vi "acq_eeg_read.vi"(7 "Marker Queue":refnum<queue>, 8 "error in (no error)":errorcluster, 10 "variant in":variant, 11 "eeg_device":T1) -> (0 "error out":errorcluster, 1 "Next Acq State":string, 2 "Variant out":variant, 3 "eeg samples":dbl[][](array[numeric]), 5 "Marker Queue Out":refnum<queue>)   [LabVIEW 2013]
uses:
  <vilib>/NIOSC/Address Space Node.ctl
  gui/type_def/device.ctl
  <vilib>/NI/Emotiv Toolkit/Emotiv Task.lvclass
  <vilib>/NI/Emotiv Toolkit/Utilities/EE DataChannels_enum.ctl
  <vilib>/OpenBCI/Comm Protocol/Control Def/openbci_device.ctl
  <vilib>/OpenBCI/Comm Protocol/Control Def/channel_count.ctl
  gui/type_def/file_stream.ctl
  <vilib>/NIOSC/Argument to Float32 Data.vi
  <vilib>/NIOSC/Generate Error.vi
  <vilib>/NI/LabVIEW - NeuroSky Driver/NeuroSky Driver/ThinkGear Read/ThinkGear MultiSample Read Raw.vi
  <vilib>/NIOSC/NI_OSC.lvlib
  <vilib>/NI/LabVIEW - NeuroSky Driver/NeuroSky Driver.lvlib
panel:
  out "Livesign Msg":bool
  out "ECG Chart":u32[](graph)
  out "Acc Chart":dbl[][](graph)
  out "Respiration Chart":u32[](graph)
  in  "NeuroSky Task Out":T2
  in  "muse cluster out":T4
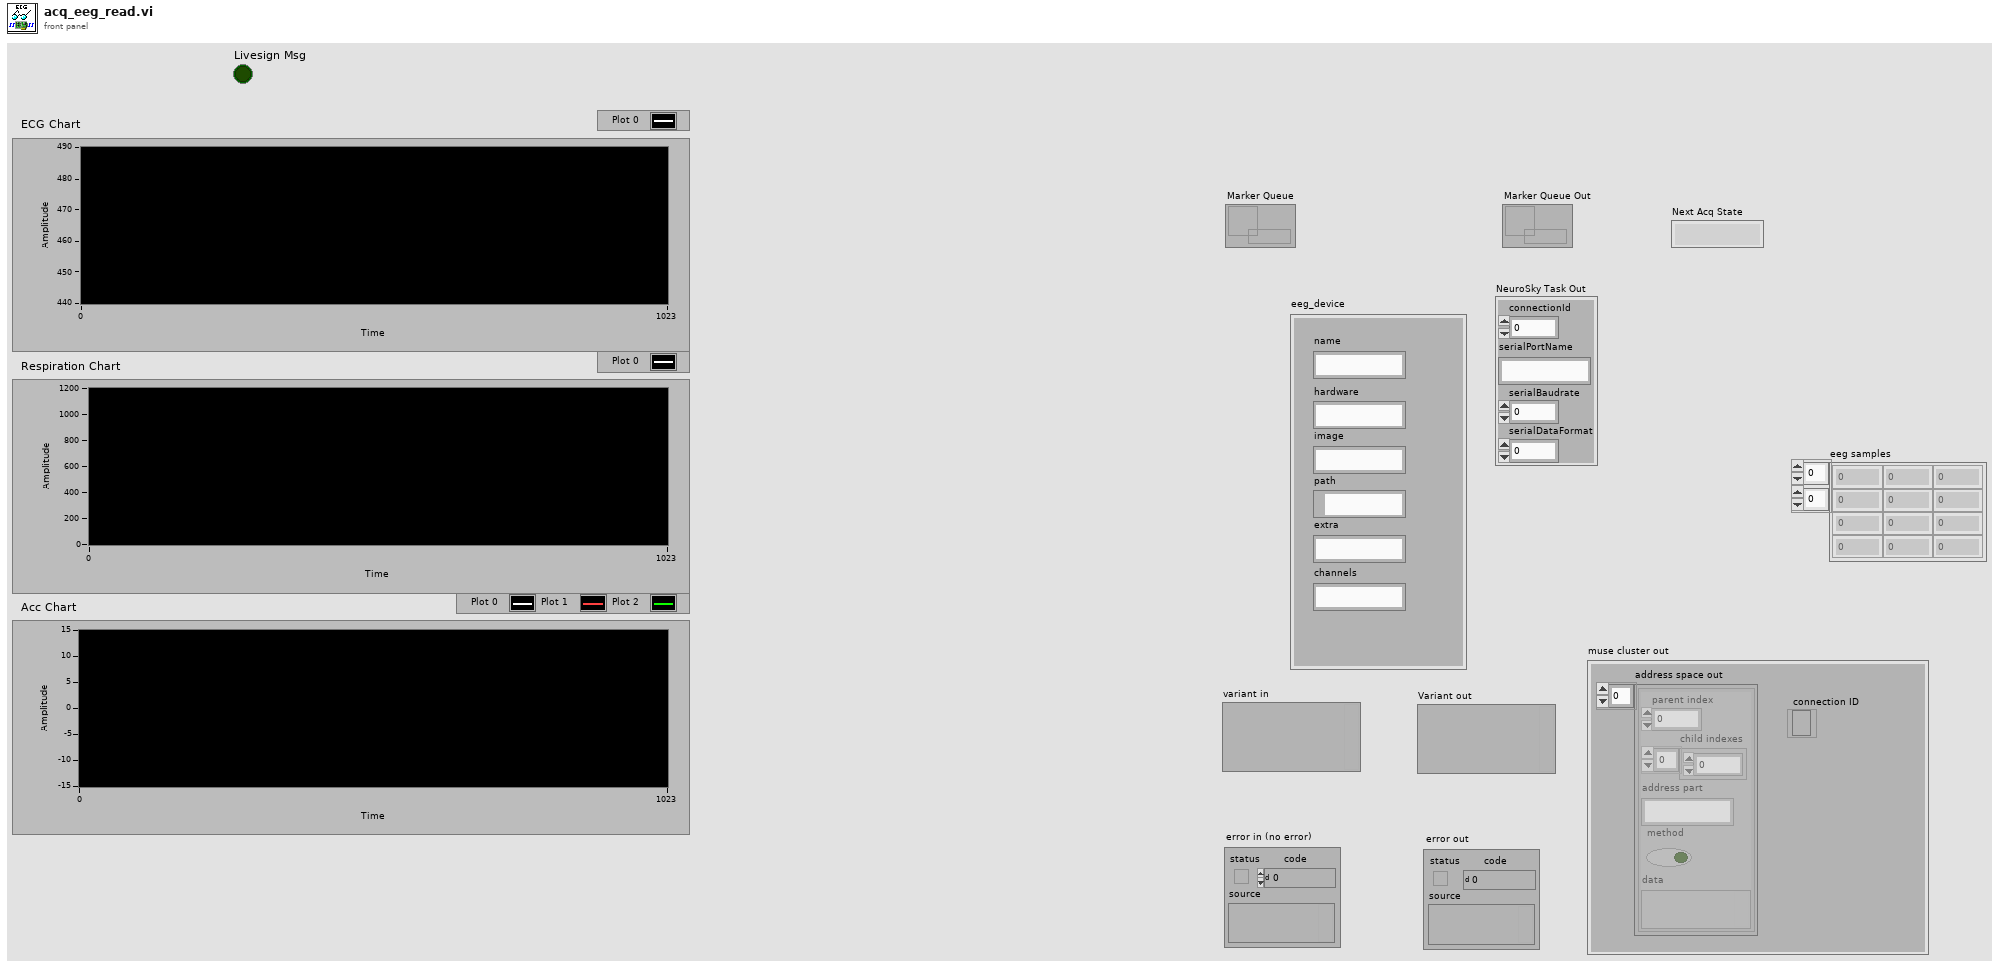
[diagram p1: front panel]
types:
  T1 = typedef "device.ctl" = cluster{"name":string, "hardware":string, "image":string, "path":path, "extra":string, "channels":string}
  T2 = cluster{"connectionId":i32, "serialPortName":string, "serialBaudrate":i32, "serialDataFormat":i32}
  T3 = typedef "NI_OSC.lvlib/Address Space Node.ctl" = cluster{"parent index":i32, "child indexes":i32[], "address part":string, "method":bool, "data":variant}
  T4 = cluster{"address space out":T3[], "connection ID":refnum<k5>}
  T5 = typedef "Emotiv Task.lvclass/EE DataChannels_enum.ctl" = enum8{"ED_COUNTER", "ED_INTERPOLATED", "ED_RAW_CQ", "ED_AF3", "ED_F7", "ED_F3", "ED_FC5", "ED_T7", "ED_P7", "ED_O1", "ED_O2", "ED_P8", "ED_T8", "ED_FC6", "ED_F4", "ED_F8", "ED_AF4", "ED_GYROX", "ED_GYROY", "ED_TIMESTAMP", "ED_ES_TIMESTAMP", "ED_FUNC_ID", "ED_FUNC_VALUE", "ED_MARKER", "ED_SYNC_SIGNAL"}
  T6 = typedef "openbci_device.ctl" = cluster{"COM port":refnum<visa-resource-name>, "n_ch (8)":T7, "delay_tx":u32}
  T7 = typedef "channel_count.ctl" = enum16{"8 Channels", "16 Channels"}
  T8 = typedef "file_stream.ctl" = cluster{"timestamp":timestamp, "data (2D array)":dbl[][], "Reading?":bool}
  T9 = typedef "NI_OSC.lvlib/Method Dispatching Info.ctl" = cluster{"method address":string, "message":string, "message timetag":u64, "data":variant}
  T10 = typedef "NI_OSC.lvlib/Argument.ctl" = cluster{"argument":string, "type tag":string}
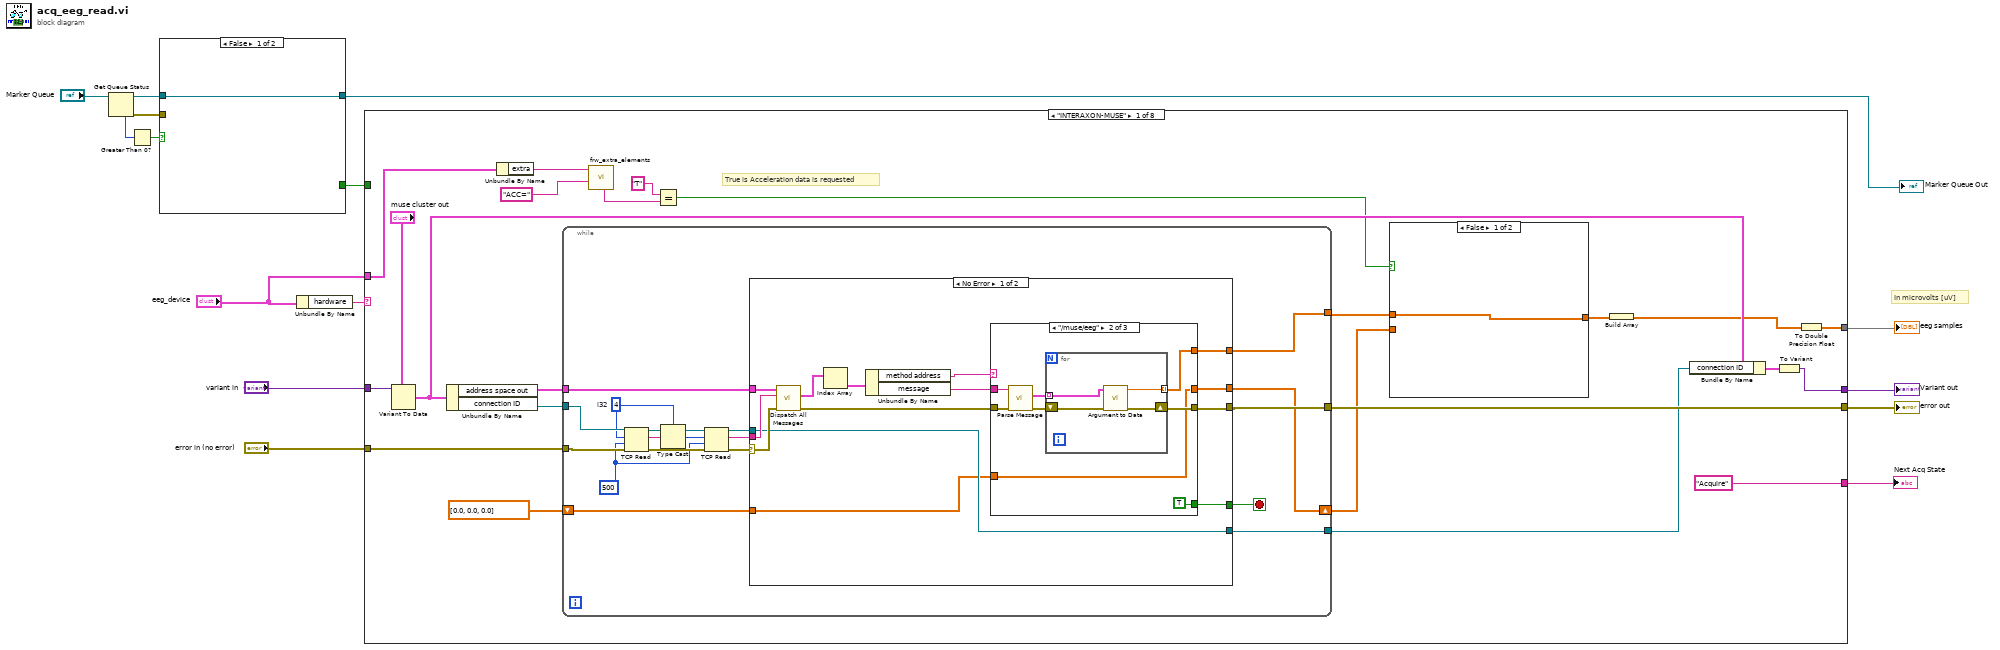
[diagram p0: block diagram]
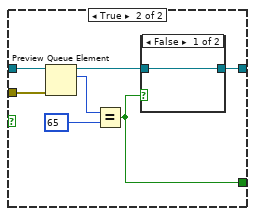
[diagram p2: hidden frame]
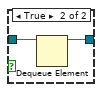
[diagram p3: hidden frame]
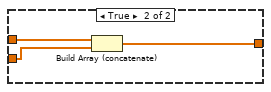
[diagram p4: hidden frame]
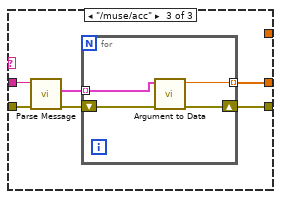
[diagram p6: hidden frame]
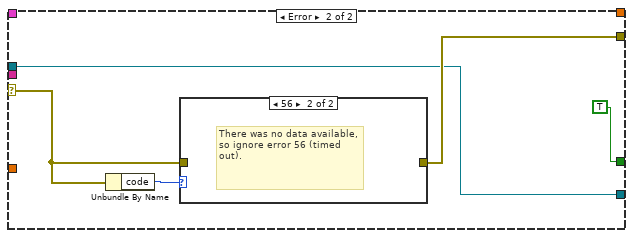
[diagram p7: hidden frame]
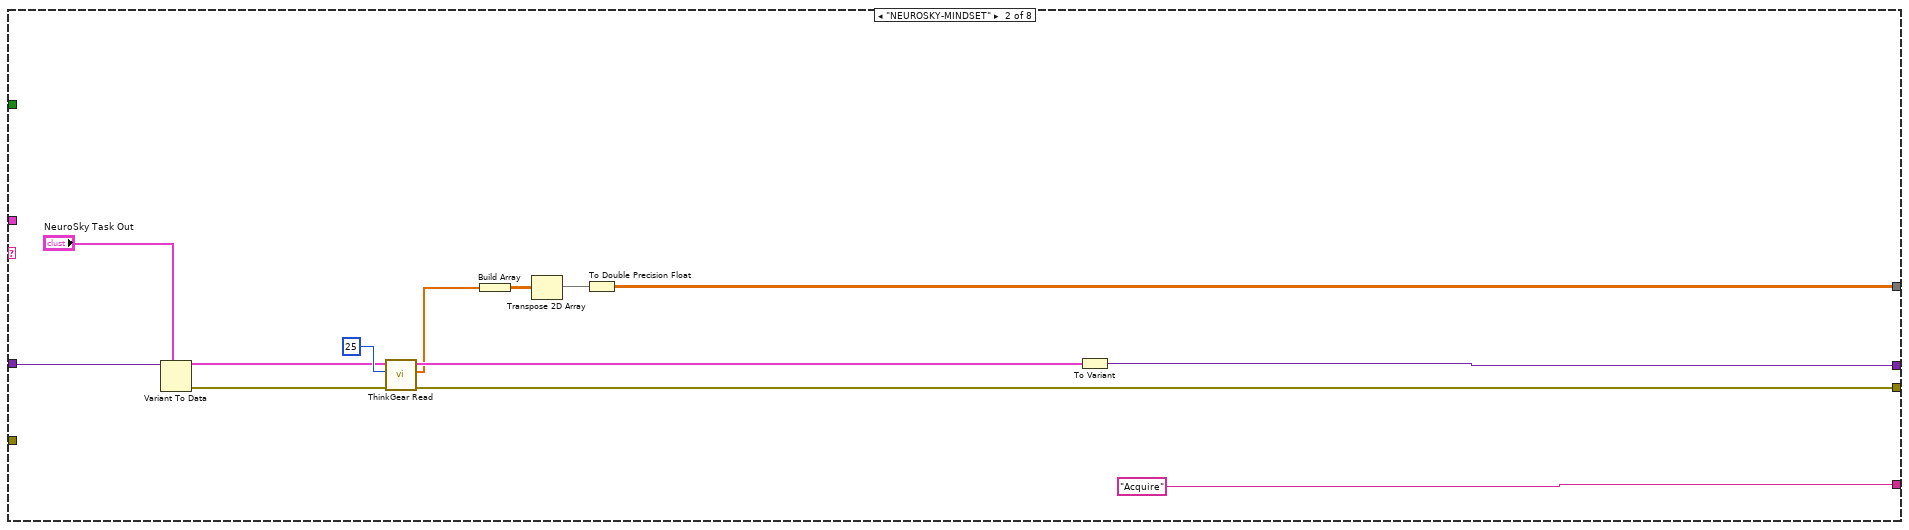
[diagram p9: hidden frame]
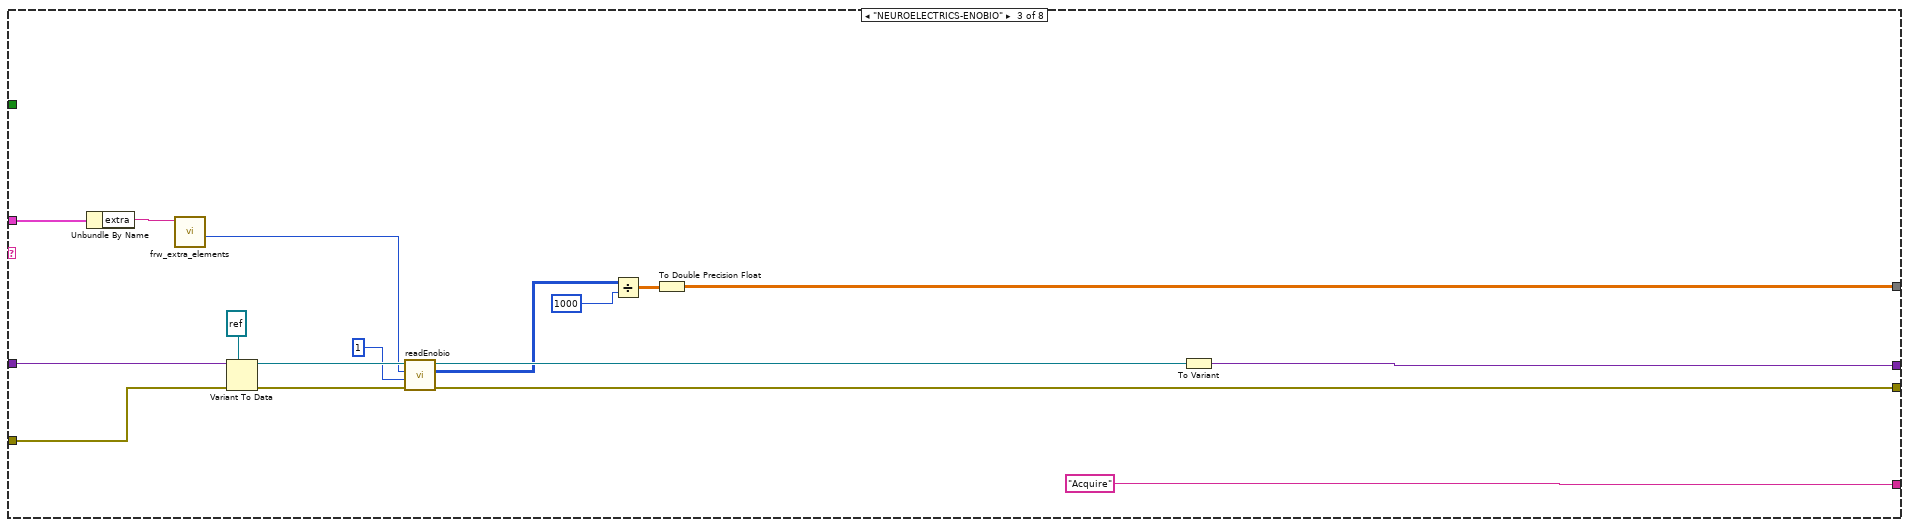
[diagram p10: hidden frame]
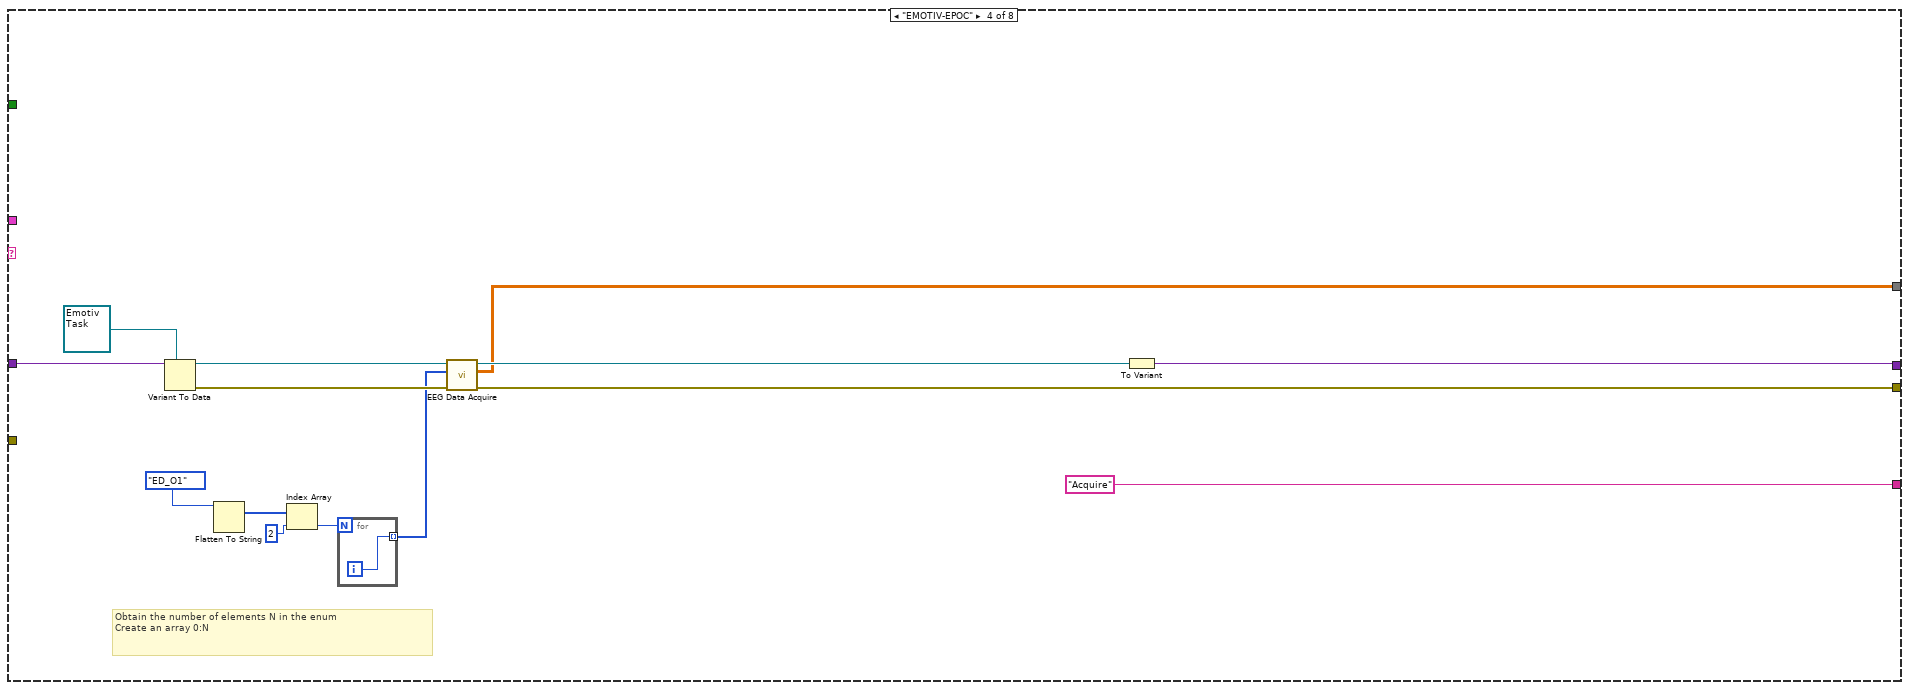
[diagram p11: hidden frame]
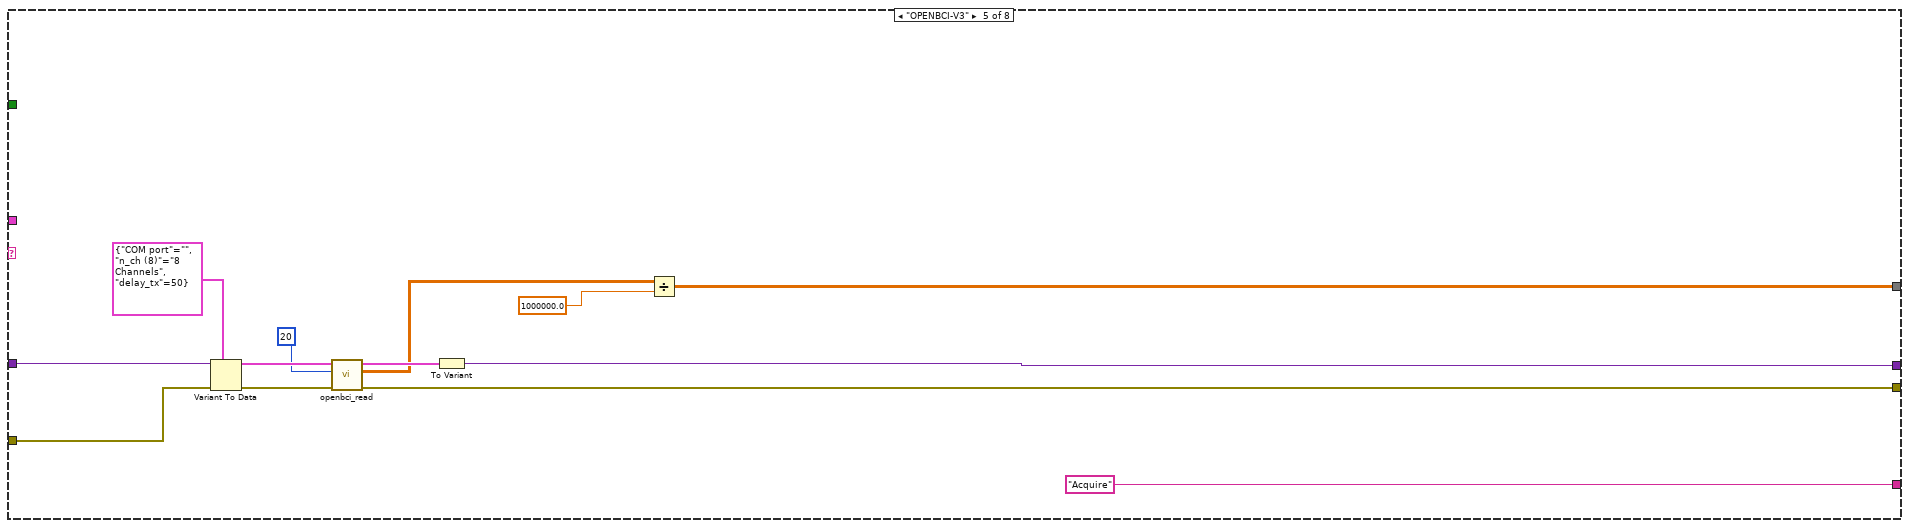
[diagram p12: hidden frame]
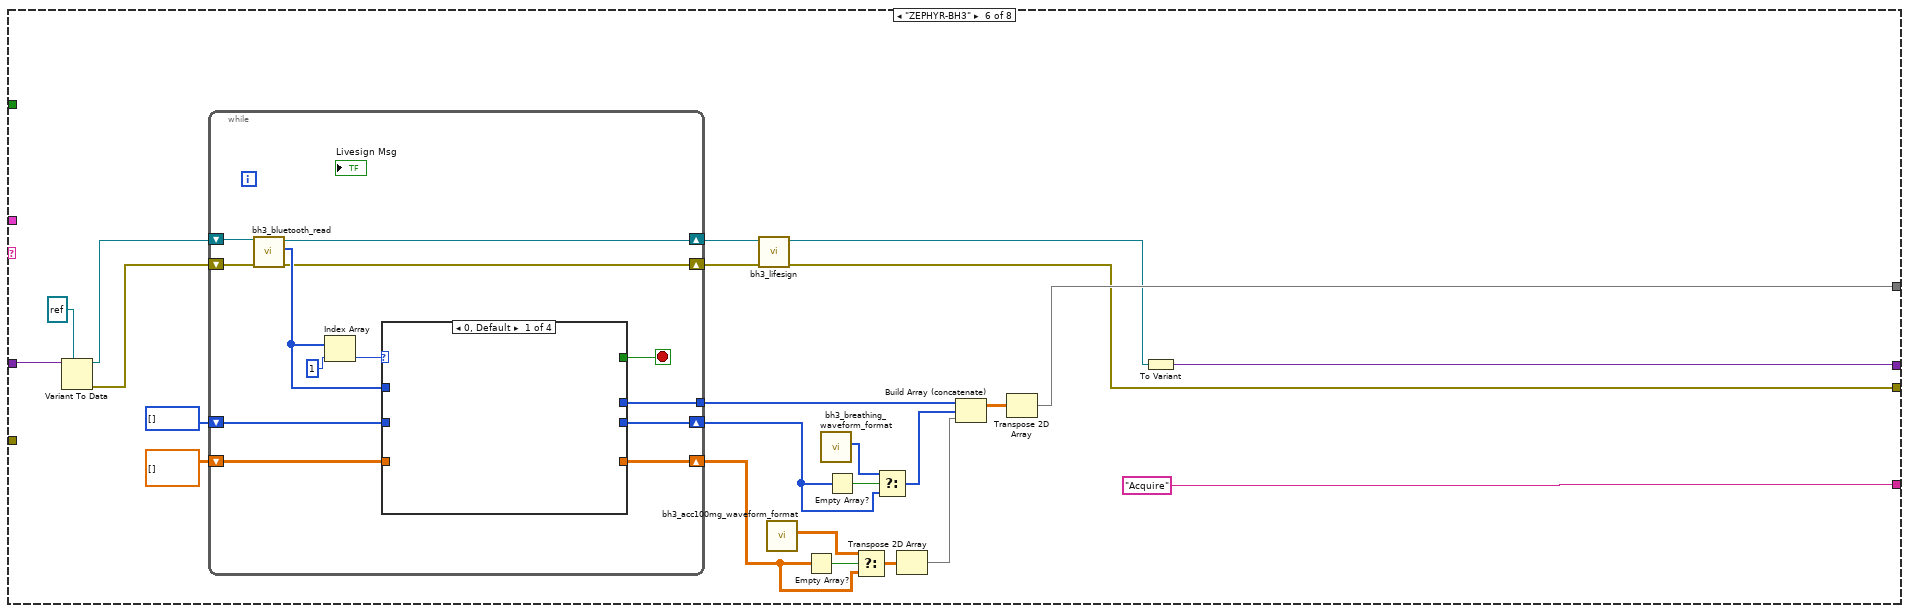
[diagram p13: hidden frame]
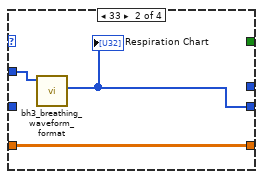
[diagram p14: hidden frame]
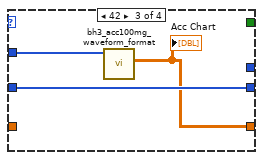
[diagram p15: hidden frame]
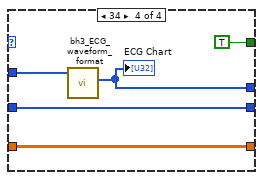
[diagram p16: hidden frame]
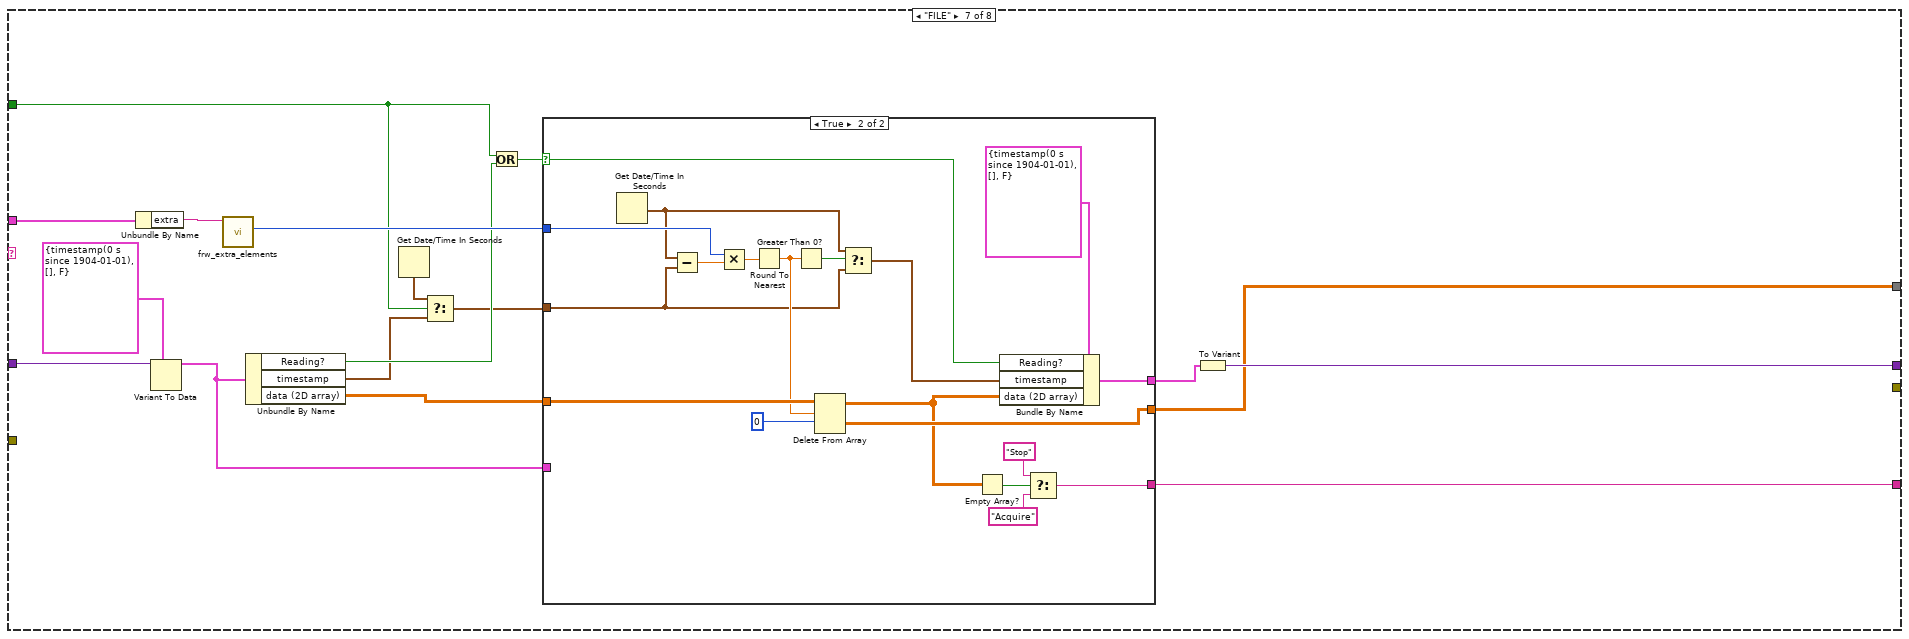
[diagram p17: hidden frame]
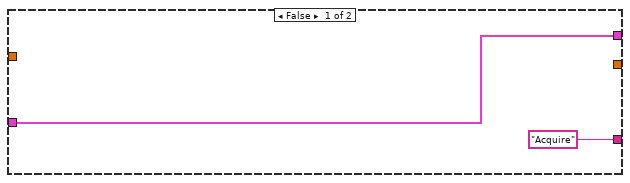
[diagram p18: hidden frame]
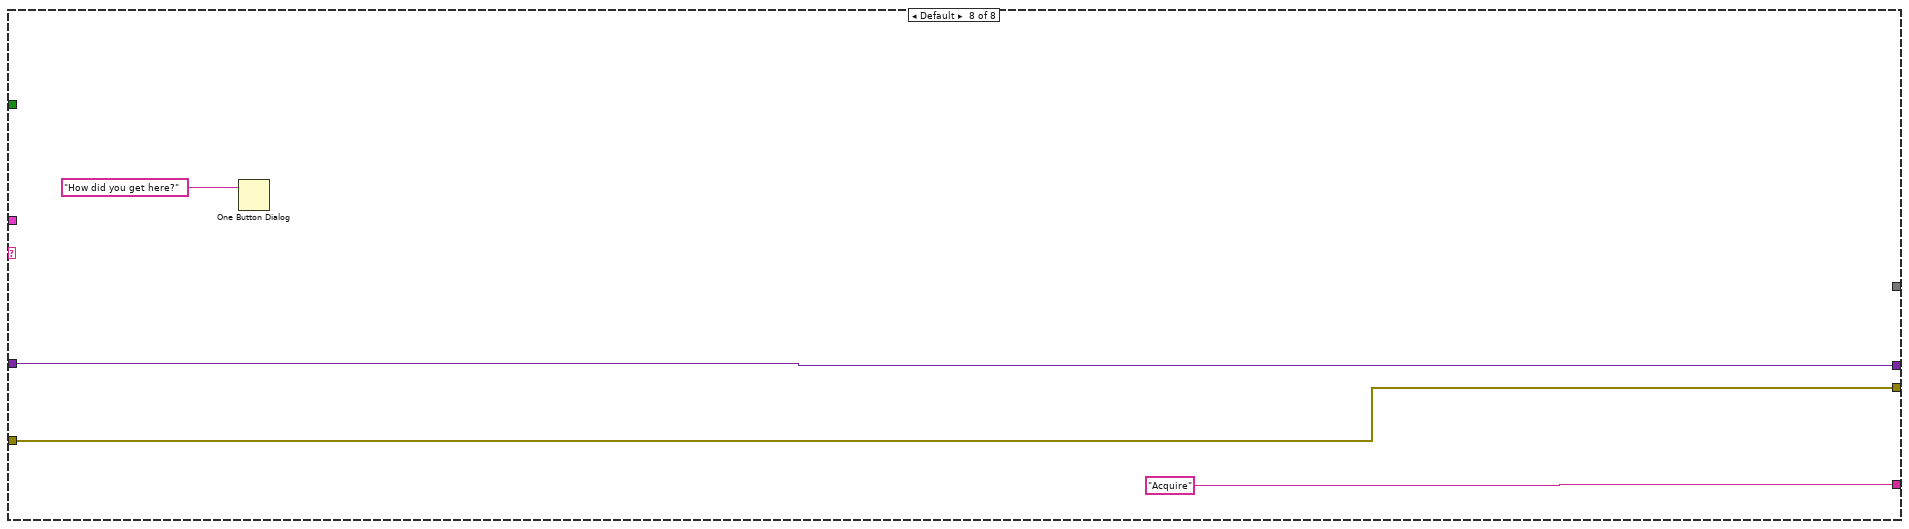
[diagram p19: hidden frame]
diagram:
  # "In microvolts [uV]"
  n1 = Get Queue Status(queue="Marker Queue") -> (queue out=w6:refnum<queue>, error out=w7:errorcluster, # elements in queue=w4:i32)  [unwired: 2 in, 5 out]
  n2 = Greater Than 0?(x=w4) -> (x > 0?=w5:bool)
  n3 = case shown="False" w5 {
    tunnel: w6 -> [w16 w23]
    tunnel: w7 -> [_ w22]
    tunnel: [w16 w19] -> w2
    tunnel: [_ w17] -> w1
    frame False {
    }
    frame True {
      n4 = Preview Queue Element(queue=w23, error in (no error)=w22) -> (queue out=w18:refnum<queue>, element=w21:u8)  [unwired: 1 in, 2 out]
      n5 = Equal?(x=w21, y=u8 65) -> (x = y?=w17:bool)
      n6 = case shown="False" w17 {
        tunnel: [w24 w26] -> w19
        tunnel: w18 -> [w24 w25]
        frame False {
        }
        frame True {
          n7 = Dequeue Element(queue=w25) -> (queue out=w26:refnum<queue>)  [unwired: 2 in, 3 out]
        }
      }
    }
  }
  "Marker Queue Out" <- w2
  n8 = Unbundle By Name("eeg_device") -> ("hardware"=w15:string)
  n9 = case shown="\"INTERAXON-MUSE\"" w15 {
    tunnel: "eeg_device" -> [w39 _ w131 _ _ _ w235 _]
    tunnel: "error in (no error)" -> [w46 _ w143 _ w169 _ _ w263]
    tunnel: [w45 w123 w137 w151 w165 w175 _ w263] -> w9
    tunnel: [w30 w117 w136 w147 w161 w179 w232 _] -> w13
    tunnel: "variant in" -> [w49 w128 w144 w148 w172 w183 w238 w262]
    tunnel: [w42 w122 w139 w150 w166 w180 w236 w262] -> w11
    tunnel: ["Acquire" ("Message") "Acquire" ("Message") "Acquire" ("Message") "Acquire" ("Message") "Acquire" ("Message") "Acquire" ("Message") w227 "Acquire" ("Message")] -> w8
    tunnel: w1 -> [_ _ _ _ _ _ w226 _]
    frame "INTERAXON-MUSE" {
      # "True is Acceleration data is requested"
      n10 = Variant To Data(type="muse cluster out", Variant=w49) -> (data=w41:T4)  [unwired: 1 in, 1 out]
      n11 = Unbundle By Name(w41) -> ("address space out"=w48:T3[], "connection ID"=w47:refnum<k5>)
      n12 = Unbundle By Name(w39) -> ("extra"=w38:string)
      n13 = while {
        tunnel: w48 -> [w71]
        tunnel: w47 -> [w70]
        tunnel: w46 -> [w61]
        tunnel: [w60] -> w45
        tunnel: [w59] -> w44
        tunnel: [w57] -> w32
        shift-right: [w55] -> w31
        shift-left: sgl[] [0.0, 0.0, 0.0] -> [w54]
        stop <- w56 stop-if-true
        w58 = 500 ("timeout ms (25000)")
        w62 = 4  # i32
        n14 = TCP Read(connection ID=w70, bytes to read=w62, error in (no error)=w61, 9:w58) -> (connection ID out=w67:refnum<k5>, data out=w63:string, error out=w69:errorcluster)  [unwired: 1 in]
        n15 = Type Cast(type=w62, x=w63) -> (*(type *) &x=w64:i32)
        n16 = TCP Read(connection ID=w67, bytes to read=w64, error in (no error)=w69, 9:w58) -> (connection ID out=w66:refnum<k5>, data out=w65:string, error out=w68:errorcluster)  [unwired: 1 in]
        n17 = case shown="No Error" w68 {
          selector: w68 -> [w84 w113]
          tunnel: w66 -> [w79 w111]
          tunnel: [w79 w111] -> w59
          tunnel: [w82 w112] -> w60
          tunnel: w65 -> [w81 _]
          tunnel: w71 -> [w85 _]
          tunnel: [w80 _] -> w57
          tunnel: [w74 _] -> w55
          tunnel: [w73 TRUE] -> w56
          tunnel: w54 -> [w72 _]
          frame No Error {
            n18 = call <vilib>:"Dispatch All Messages.vi"("error in"=w84, "packet"=w81, "address space in"=w85) -> ("error out"=w83:errorcluster, "method dispatching info"=w76:T9[])  [unwired: 6 in, 1 out]
            n19 = Index Array(array=w76) -> (element=w75:T9)  [unwired: 1 in]
            n20 = Unbundle By Name(w75) -> ("method address"=w78:string, "message"=w77:string)
            n21 = case shown="\"/muse/eeg\"" w78 {
              tunnel: w83 -> [w87 w95 w105]
              tunnel: [w87 w92 w101] -> w82
              tunnel: w77 -> [_ w94 w104]
              tunnel: [_ w90 _] -> w80
              tunnel: [w86 w88 w100] -> w74
              tunnel: [_ TRUE _] -> w73
              tunnel: w72 -> [w86 w88 _]
              frame Default {
              }
              frame "/muse/eeg" {
                n22 = call <vilib>:"Parse Message.vi"("error in"=w95, "message"=w94) -> ("error out"=w93:errorcluster, "arguments"=w91:T10[])  [unwired: 7 in, 1 out]
                n23 = for {
                  tunnel: w91 -> [w98] mode=indexing
                  tunnel: [w97] -> w90 mode=indexing
                  shift-right: [w96] -> w92
                  shift-left: w93 -> [w99]
                  n24 = call-poly <vilib>:"Argument to Data.vi"("error in"=w99, "float32 argument"=w98) -> ("error out"=w96:errorcluster, "float32 data"=w97:sgl)  [unwired: 8 in]
                }
              }
              frame "/muse/acc" {
                n25 = call <vilib>:"Parse Message.vi"("error in"=w105, "message"=w104) -> ("error out"=w103:errorcluster, "arguments"=w102:T10[])  [unwired: 7 in, 1 out]
                n26 = for {
                  tunnel: w102 -> [w108] mode=indexing
                  tunnel: [w107] -> w100 mode=indexing
                  shift-right: [w106] -> w101
                  shift-left: w103 -> [w109]
                  n27 = call-poly <vilib>:"Argument to Data.vi"("error in"=w109, "float32 argument"=w108) -> ("error out"=w106:errorcluster, "float32 data"=w107:sgl)  [unwired: 8 in]
                }
              }
            }
          }
          frame Error {
            n28 = Unbundle By Name(w113) -> ("code"=w114:i32)
            n29 = case shown="56" w114 {
              tunnel: w113 -> [w115 _]
              tunnel: [w115 _] -> w112
              frame Default {
              }
              frame 56 {
                # "There was no data available, so ignore error 56 (timed out)."
              }
            }
          }
        }
      }
      n30 = call "frw_extra_elements.vi"("single field"="ACC=", "string"=w38) -> ("single string"=w35:string)  [unwired: 5 in, 4 out]
      n31 = Equal?(x="T", y=w35) -> (x = y?=w33:bool)
      n32 = case shown="False" w33 {
        tunnel: [w50 w51] -> w29
        tunnel: w32 -> [w50 w53]
        tunnel: w31 -> [_ w52]
        frame False {
        }
        frame True {
          n33 = Build Array (concatenate)(w53, w52) -> (w51:sgl[])
        }
      }
      n34 = Build Array(w29) -> (w28:sgl[][])
      n35 = Bundle By Name(cluster=w41, "connection ID"=w44) -> (w43:T4)
      n36 = To Variant(anything=w43) -> (Variant=w42:variant)
      n37 = To Double Precision Float(number=w28) -> (double precision float=w30:dbl[][])
    }
    frame "NEUROSKY-MINDSET" {
      n38 = Variant To Data(type="NeuroSky Task Out", Variant=w128) -> (data=w124:T2, error out=w125:errorcluster)  [unwired: 1 in]
      n39 = call-poly <vilib>:"ThinkGear Read.vi"("error in (no error)"=w125, "Samples to Read"=25, "NeuroSky Task In"=w124) -> ("error out"=w123:errorcluster, "Data Out"=w120:sgl[], "NeuroSky Task Out"=w121:T2)  [unwired: 6 in]
      n40 = Build Array(w120) -> (w119:sgl[][])
      n41 = Transpose 2D Array(2D array=w119) -> (transposed array=w118:sgl[][])
      n42 = To Double Precision Float(number=w118) -> (double precision float=w117:dbl[][])
      n43 = To Variant(anything=w121) -> (Variant=w122:variant)
    }
    frame "NEUROELECTRICS-ENOBIO" {
      n44 = Unbundle By Name(w131) -> ("extra"=w130:string)
      n45 = call "frw_extra_elements.vi"("string"=w130) -> ("#ch"=w129:i32)  [unwired: 6 in, 4 out]
      n46 = Variant To Data(error in=w143, type=refnum<k5> refnum ("connection ID"), Variant=w144) -> (data=w142:refnum<k5>, error out=w141:errorcluster)
      n47 = call "readEnobio.vi"("error in (no error)"=w141, "nSamples"=1, "nChannels"=w129, "connection ID"=w142) -> ("error out"=w137:errorcluster, "output array"=w134:i32[][], "connection ID out"=w138:refnum<k5>)  [unwired: 5 in]
      n48 = Divide(x=w134, y=1000) -> (x/y=w135:dbl[][])
      n49 = To Double Precision Float(number=w135) -> (double precision float=w136:dbl[][])
      n50 = To Variant(anything=w138) -> (Variant=w139:variant)
    }
    frame "EMOTIV-EPOC" {
      # "Obtain the number of elements N in the enum\nCreate an array 0:N"
      n51 = Variant To Data(type=refnum<class "Emotiv Task.lvclass"> refnum ("Emotiv Task in"), Variant=w148) -> (data=w158:refnum<class "Emotiv Task.lvclass">, error out=w157:errorcluster)  [unwired: 1 in]
      n52 = Flatten To String(anything=EE_DataChannels_enum."ED_O1" ("EE_InputChannels_enum")) -> (type string=w154:i16[])  [unwired: 3 in, 2 out]
      n53 = Index Array(array=w154, index=2) -> (element=w153:i16)
      n54 = for {
        N: w153 -> [_]
        tunnel: [w160] -> w152 mode=indexing
        i -> [w160]
      }
      n55 = call <vilib>:"EEG Data Acquire.vi"("error in (no error)"=w157, "channel_array"=w152, "Emotiv Task in"=w158) -> ("error out"=w151:errorcluster, "EEG data"=w147:dbl[][], "Emotiv Task out"=w149:refnum<class "Emotiv Task.lvclass">)  [unwired: 5 in, 1 out]
      n56 = To Variant(anything=w149) -> (Variant=w150:variant)
    }
    frame "OPENBCI-V3" {
      n57 = Variant To Data(error in=w169, type=T6 {"COM port"="", "n_ch (8)"=enum."8 Channels", "delay_tx"=50} ("OBCI dev in"), Variant=w172) -> (data=w171:T6, error out=w170:errorcluster)
      n58 = call <vilib>:"openbci_read.vi"("error in"=w170, "N samples (2)"=20, "OBCI dev in"=w171) -> ("error out"=w165:errorcluster, "EEG data"=w163:dbl[][], "OBCI dev out"=w167:T6)  [unwired: 5 in, 1 out]
      n59 = To Variant(anything=w167) -> (Variant=w166:variant)
      n60 = Divide(x=w163, y=1000000.0) -> (x/y=w161:dbl[][])
    }
    frame "ZEPHYR-BH3" {
      n61 = Variant To Data(type=refnum<k31> refnum ("bt connection ID out"), Variant=w183) -> (data=w182:refnum<k31>, error out=w181:errorcluster)  [unwired: 1 in]
      n62 = while {
        shift-right: [w202] -> w177
        shift-left: w182 -> [w205]
        shift-right: [w203] -> w178
        shift-left: w181 -> [w204]
        tunnel: [w206] -> w185
        shift-right: [w201] -> w189
        shift-left: u32[] [] ("breathing data") -> [w200]
        shift-right: [w199] -> w193
        shift-left: dbl[][] [] ("acc (G)") -> [w198]
        stop <- w207 stop-if-true
        n63 = call <vilib>:"bh3_bluetooth_read.vi"("error in (no error)"=w204, "bt connection ID in"=w205) -> ("error out"=w203:errorcluster, "response byte array"=w208:u8[], "bt connection ID out"=w202:refnum<k31>)  [unwired: 7 in]
        n64 = Index Array(array=w208, index=1) -> (element=w210:u8)
        n65 = case shown="0, Default" w210 {
          tunnel: w208 -> [_ w213 w216 w221]
          tunnel: [_ _ _ TRUE] -> w207
          tunnel: [_ _ _ w219] -> w206
          tunnel: [_ w212 w215 w218] -> w201
          tunnel: w200 -> [_ _ w215 w218]
          tunnel: [_ w211 w214 w217] -> w199
          tunnel: w198 -> [_ w211 _ w217]
          frame 0, Default {
          }
          frame 33 {
            n66 = call <vilib>:"bh3_breathing_waveform_format.vi"("Breathing Waveform Packet"=w213) -> ("breathing data"=w212:u32[])  [unwired: 5 in, 5 out]
            "Respiration Chart" <- w212
          }
          frame 42 {
            n67 = call <vilib>:"bh3_acc100mg_waveform_format.vi"("Acc 100mg Waveform Packet"=w216) -> ("acc (G)"=w214:dbl[][])  [unwired: 5 in, 5 out]
            "Acc Chart" <- w214
          }
          frame 34 {
            n68 = call <vilib>:"bh3_ECG_waveform_format.vi"("ECG Waveform Packet"=w221) -> ("ECG data"=w219:u32[])  [unwired: 5 in, 5 out]
            "ECG Chart" <- w219
          }
        }
      }
      n69 = call <vilib>:"bh3_lifesign.vi"("error in (no error)"=w178, "bt connection ID in"=w177) -> ("error out"=w175:errorcluster, "bt connection ID out"=w176:refnum<k31>)  [unwired: 8 in]
      n70 = call <vilib>:"bh3_acc100mg_waveform_format.vi"() -> ("acc (G)"=w194:dbl[][])  [unwired: 6 in, 5 out]
      n71 = Empty Array?(array=w193) -> (empty?=w192:bool)
      n72 = call <vilib>:"bh3_breathing_waveform_format.vi"() -> ("breathing data"=w187:u32[])  [unwired: 6 in, 5 out]
      n73 = Empty Array?(array=w189) -> (empty?=w188:bool)
      n74 = Select(t=w194, s=w192, f=w193) -> (s? t:f=w196:dbl[][])
      n75 = Select(t=w187, s=w188, f=w189) -> (s? t:f=w190:u32[])
      n76 = Transpose 2D Array(2D array=w196) -> (transposed array=w197:dbl[][])
      n77 = Build Array (concatenate)(w185, w190, w197) -> (w186:dbl[][])
      n78 = Transpose 2D Array(2D array=w186) -> (transposed array=w179:dbl[][])
      n79 = To Variant(anything=w176) -> (Variant=w180:variant)
    }
    frame "FILE" {
      n80 = Unbundle By Name(w235) -> ("extra"=w234:string)
      n81 = Variant To Data(type=T8 {"timestamp"=timestamp(0 s since 1904-01-01), "data (2D array)"=[], "Reading?"=FALSE} ("output cluster"), Variant=w238) -> (data=w222:T8)  [unwired: 1 in, 1 out]
      n82 = call "frw_extra_elements.vi"("string"=w234) -> ("fs"=w233:i32)  [unwired: 6 in, 4 out]
      n83 = Unbundle By Name(w222) -> ("Reading?"=w228:bool, "timestamp"=w225:timestamp, "data (2D array)"=w230:dbl[][])
      n84 = Get Date/Time In Seconds() -> (seconds since 1Jan1904=w223:timestamp)
      n85 = Select(t=w223, s=w226, f=w225) -> (s? t:f=w224:timestamp)
      n86 = Or(x=w226, y=w228) -> (x .or. y?=w229:bool)
      n87 = case shown="True" w229 {
        selector: w229 -> [_ w252]
        tunnel: w233 -> [_ w258]
        tunnel: [_ w256] -> w232
        tunnel: [w239 w254] -> w231
        tunnel: w230 -> [_ w253]
        tunnel: ["Acquire" ("Message") w246] -> w227
        tunnel: w224 -> [_ w241]
        tunnel: w222 -> [w239 _]
        frame False {
        }
        frame True {
          n88 = Get Date/Time In Seconds() -> (seconds since 1Jan1904=w244:timestamp)
          n89 = Subtract(x=w244, y=w241) -> (x-y=w259:dbl)
          n90 = Multiply(x=w258, y=w259) -> (x*y=w257:dbl)
          n91 = Round To Nearest(number=w257) -> (nearest integer value=w242:dbl)
          n92 = Greater Than 0?(x=w242) -> (x > 0?=w245:bool)
          n93 = Delete From Array(array=w253, length=w242, index (row)=0) -> (deleted portion=w256:dbl[][], array with subset deleted=w250:dbl[][])  [unwired: 1 in]
          n94 = Select(t=w244, s=w245, f=w241) -> (s? t:f=w243:timestamp)
          n95 = Empty Array?(array=w250) -> (empty?=w248:bool)
          n96 = Bundle By Name(cluster=T8 {"timestamp"=timestamp(0 s since 1904-01-01), "data (2D array)"=[], "Reading?"=FALSE} ("output cluster"), "Reading?"=w252, "timestamp"=w243, "data (2D array)"=w250) -> (w254:T8)
          n97 = Select(t="Stop" ("Message"), s=w248, f="Acquire" ("Message")) -> (s? t:f=w246:string)
        }
      }
      n98 = To Variant(anything=w231) -> (Variant=w236:variant)
    }
    frame Default {
      n99 = One Button Dialog(message="How did you get here?") -> ()  [unwired: 1 in, 1 out]
    }
  }
  "error out" <- w9
  "eeg samples" <- w13
  "Variant out" <- w11
  "Next Acq State" <- w8
